vi "Mono_SetWavelength-writeCommand.vi"(8 "error in (no error) 2":errorcluster, 9 "Wavelength":dbl, 10 "Mono Wait time (ms)":u32, 11 "CmdLib In":refnum<k24>) -> (0 "error out 2":errorcluster, 1 "Wavelength Set":bool=TRUE, 3 "CmdLib Out":refnum<k24>)   [LabVIEW 2023]
uses:
  E:/Old PC/desktop/Sensitive EQE Stuff/S-EQE (YJ)/Mono vi (YJ)/Cornerstone.dll
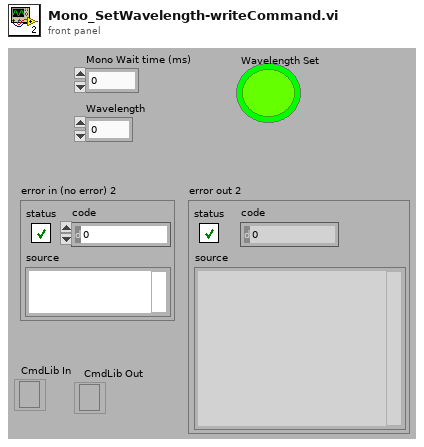
[diagram p1: front panel]
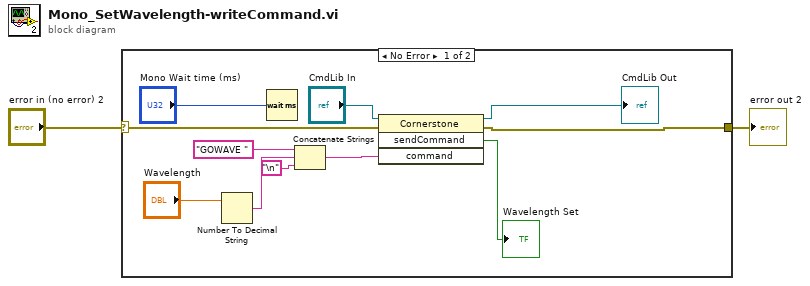
[diagram p0: block diagram]
diagram:
  n1 = case shown="No Error" "error in (no error) 2" {
    selector: "error in (no error) 2" -> [w13 w14]
    tunnel: [w3 w14] -> w1
    frame No Error {
      n2 = Number To Decimal String(number="Wavelength") -> (decimal integer string=w7:string)  [unwired: 1 in]
      n3 = Wait (ms)(milliseconds to wait="Mono Wait time (ms)") -> ()  [unwired: 1 out]
      n4 = Concatenate Strings("GOWAVE ", w7, "\n") -> (w5:string)
      n5 = invoke class="Cornerstone" method="sendCommand"(reference="CmdLib In", error in=w13, "command"=w5) -> (reference out=→"CmdLib Out":refnum<k24>, error out=w3:errorcluster, "sendCommand"=→"Wavelength Set":bool)  [unwired: 1 in, 1 out]
    }
    frame Error {
    }
  }
  "error out 2" <- w1
